vi "ECS - Scopes - DI4 Scope.vi"(11 "FPGA Ref":T1) -> ()   [LabVIEW 2015, in "ECS-RT.lvlib"]
uses:
  ECS-RT.lvlib
  Typedefs/FPGA Refs/Generic FPGA Ref.ctl
  <vilib>/Platform/TimedLoop/XDataNode/timing_clust.ctl
  <vilib>/Platform/TimedLoop/XDataNode/nitl_modes.ctl
  <vilib>/Platform/TimedLoop/XDataNode/wakeup.ctl
  <vilib>/Utility/error.llb/Error Cluster From Error Code.vi
  <vilib>/rvi/errors/niLvFpgaAdjustHostInterfaceError.vi
  Globals/DIScope Globals.vi
  <vilib>/rvi/interface/nirviReadWriteControl/nirviReadWriteControl.xnode
  <vilib>/Platform/TimedLoop/XDataNode/XDataNode.xnode
  <vilib>/Platform/TimedLoop/XDataNode/XDNodeRunTimeDep.lvlib
  <vilib>/rvi/interface/Simulation/niFpgaSimulationCallBeginRW.vi
  NiFpgaLv.dll
  ECS-Shared.lvlib
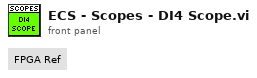
[diagram p1: front panel]
types:
  T1 = typedef "ECS-Shared.lvlib/Generic FPGA Ref.ctl" = refnum<k20>
  T2 = typedef "XDNodeRunTimeDep.lvlib/timing_clust.ctl" = cluster{"Expected End [f-1]":u64, "Actual End [f-1]":u64, "Finished Late? [f-1]":bool, "Expected End [i-1]":u64, "Actual End [i-1]":u64, "Finished Late? [i-1]":bool, "Expected Start [i]":u64, "Actual Start [i]":u64, "Expected Start [f]":u64, "Actual Start [f]":u64, "Source Name":string, "Structure Name":string, "Period":i64, "Deadline":i64, "Offset":i64, "Start":i64, "Priority":i32, "Timeout":i32, "Mode":T3, "Wakeup Reason":T4, "Error":errorcluster, "Source Type":string, "Secondary Source Type":string, "Global End Time":u64, "Global Start Time":u64, "Frame Duration":u64, "Iteration Duration":u64, "Assigned CPU":i32, "I/O Scan Engine Mode":u32}
  T3 = typedef "XDNodeRunTimeDep.lvlib/nitl_modes.ctl" = enum32{"No Change", "Process missed periods, maintain original phase", "Discard missed periods, maintain original phase", "Process missed periods, ignore original phase", "Discard missed periods, ignore original phase"}
  T4 = typedef "XDNodeRunTimeDep.lvlib/wakeup.ctl" = enum32{"Normal", "Aborted", "Asynchronous wakeup", "Timing source error", "Timed loop error", "Timeout"}
  T5 = cluster{"Element":u32, "Timed Out?":bool, "Elements Left":u32}
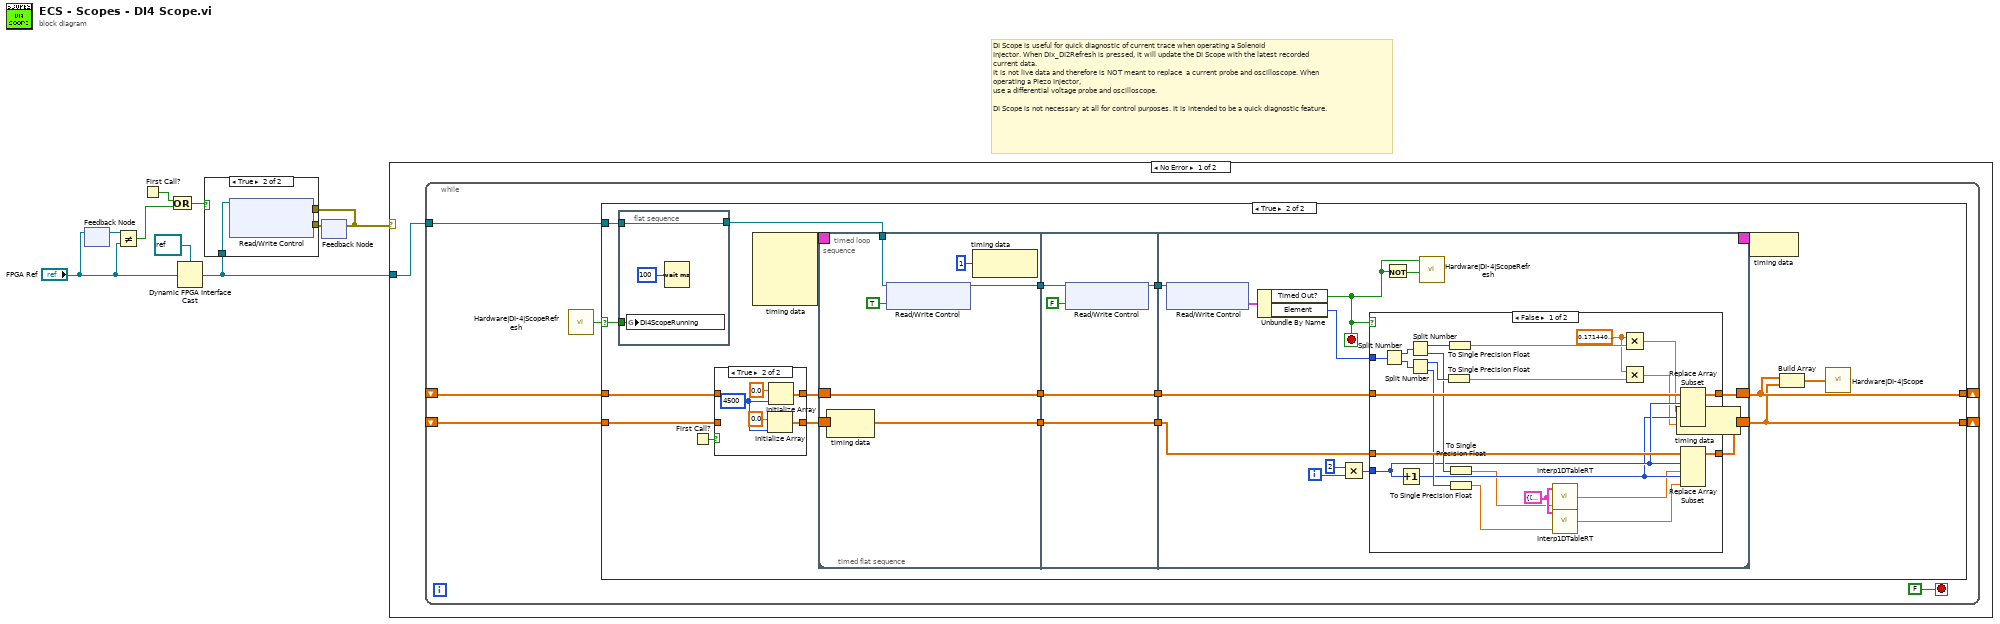
[diagram p0: block diagram]
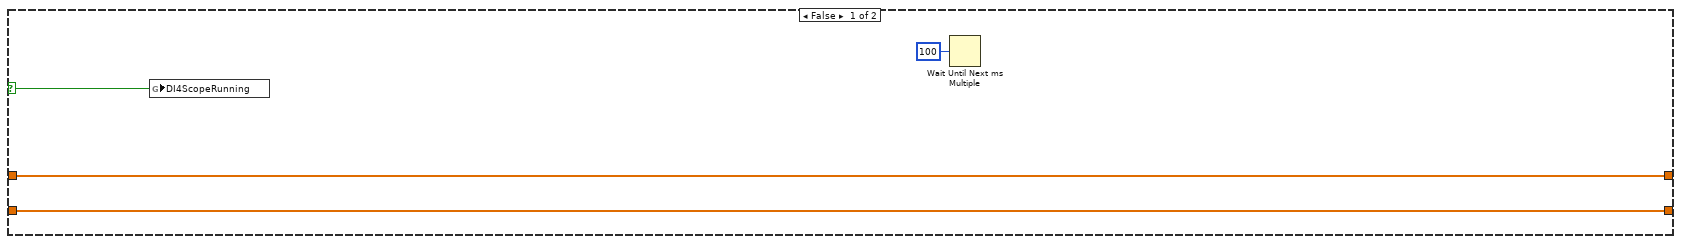
[diagram p3: hidden frame]
diagram:
  # "DI Scope is useful for quick diagnostic of current trace when operating a Solenoid\nInjector. When DIx_DI2Refresh is pressed, it will update the DI Scope with the latest recorded current data.\nIt is not live data and therefore is NOT meant to replace  a current probe and oscilloscope. When operating a Piezo Injector,\nuse a differential voltage probe and oscilloscope. \n\nDI Scope is not necessary at all for control purposes. It is intended to be a quick diagnostic feature."
  n1 = feedback #1() -> (w6:T1)  [unwired: 1 in]
  n2 = feedback-in #1("FPGA Ref") -> ()
  n3 = Not Equal?(x=w6, y="FPGA Ref") -> (x != y?=w5:bool)
  n4 = First Call?() -> (First Call?: T/F=w7:bool)
  n5 = Or(x=w7, y=w5) -> (x .or. y?=w8:bool)
  n6 = Dynamic FPGA Interface Cast(Session In=refnum<k20> refnum ("DI4 Scope"), Type="FPGA Ref") -> (Session Out=w3:refnum<k20>)
  n7 = feedback #2() -> (w9:errorcluster)  [unwired: 1 in]
  n8 = case shown="True" w8 {
    tunnel: [w10 w12] -> w4
    tunnel: w9 -> [w10 _]
    tunnel: w3 -> [_ w11]
    frame False {
    }
    frame True {
      n9 = xnode "Read/Write Control"("FPGA VI Reference In"=w11) -> ("error out"=w12:errorcluster)  [unwired: 2 in, 2 out]
    }
  }
  n10 = feedback-in #2(w4) -> ()
  n11 = case shown="No Error" w4 {
    tunnel: w3 -> [w13 _]
    frame No Error {
      n12 = while {
        shift-right: [w18] -> _
        shift-left: _ -> [w20]
        shift-right: [w17] -> _
        shift-left: _ -> [w19]
        tunnel: w13 -> [w16]
        stop <- FALSE stop-if-true
        n13 = call "Hardware|DI-4|ScopeRefresh"() -> ("Value"=w15:bool)
        n14 = case shown="True" w15 {
          selector: w15 -> [w22 w28]
          tunnel: w20 -> [w24 w35]
          tunnel: w19 -> [w23 w34]
          tunnel: [w24 w33] -> w18
          tunnel: [w23 w29] -> w17
          tunnel: w16 -> [_ w27]
          frame False {
            n15 = global write "DIScope Globals.vi" "DI4ScopeRunning"(w22) -> ()
            n16 = Wait Until Next ms Multiple(millisecond multiple=u32 100) -> ()  [unwired: 1 out]
          }
          frame True {
            n17 = flat-sequence {
              tunnel: w28 -> [w40]
              tunnel: [w38] -> w26
              tunnel: w27 -> [w38]
              frame #0 {
                n18 = global write "DIScope Globals.vi" "DI4ScopeRunning"(w40) -> ()
                n19 = Wait (ms)(milliseconds to wait=u32 100 ("millisecond multiple")) -> ()  [unwired: 1 out]
              }
            }
            n20 = First Call?() -> (First Call?: T/F=w37:bool)
            n21 = case shown="True" w37 {
              tunnel: [w118 w122] -> w36
              tunnel: [w117 w121] -> w32
              tunnel: w35 -> [w118 _]
              tunnel: w34 -> [w117 _]
              frame False {
              }
              frame True {
                w119 = 4500 ("dimension size")
                n22 = Initialize Array(sgl 0.0 ("element"), w119) -> (w121:sgl[])
                n23 = Initialize Array(sgl 0.0 ("element"), w119) -> (w122:sgl[])
              }
            }
            n24 = node-c288() -> (w31:T2)  [unwired: 4 in]
            n25 = timed-loop "Timed Loop" {
              shift-right: [w43] -> w33
              shift-left: w36 -> [w44]
              shift-right: [w41] -> w29
              shift-left: w32 -> [w42]
              tunnel: w26 -> [w45]
              timing: w31 -> [_]
              timing-out: [_] -> w30
              i -> [w77]
              stop <- w74 stop-if-true
              n26 = timed-sequence {
                timing: _ -> [_]
                timing-out: _ -> [_]
                tunnel: w45 -> [w56]
                tunnel: w44 -> [w55]
                tunnel: [w54] -> w43
                tunnel: w42 -> [w53]
                tunnel: [w52] -> w41
                n27 = timed-flat-sequence {
                  tunnel: w53 -> [w61]
                  tunnel: w55 -> [w62]
                  tunnel: w56 -> [w59]
                  tunnel: [w62] -> w49
                  tunnel: [w61] -> w48
                  tunnel: [w60] -> w47
                  tunnel: [w71] -> w51
                  tunnel: [w70] -> w50
                  tunnel: w47 -> [w68]
                  tunnel: w48 -> [w70]
                  tunnel: w49 -> [w71]
                  tunnel: [w67] -> w46
                  tunnel: [w82] -> w54
                  tunnel: [w81] -> w52
                  tunnel: w51 -> [w85]
                  tunnel: w50 -> [w84]
                  tunnel: w46 -> [w79]
                  frame #0 {
                    n28 = xnode "Read/Write Control"("FPGA VI Reference In"=w59, "DI-4.ScopeRead"=TRUE ("DIDI2Read")) -> ("FPGA VI Reference Out"=w60:refnum<k20>)  [unwired: 1 in, 1 out]
                    n29 = node-c288(i64 1 ("Start")) -> ()  [unwired: 1 out]
                  }
                  frame #1 {
                    n30 = xnode "Read/Write Control"("FPGA VI Reference In"=w68, "DI-4.ScopeRead"=FALSE ("DIDI2Read")) -> ("FPGA VI Reference Out"=w67:refnum<k20>)  [unwired: 1 in, 1 out]
                  }
                  frame #2 {
                    n31 = xnode "Read/Write Control"("FPGA VI Reference In"=w79) -> ("DI-4.ScopeData"=w80:T5)  [unwired: 1 in, 2 out]
                    n32 = Unbundle By Name(w80) -> ("Timed Out?"=w74:bool, "Element"=w76:u32)
                    n33 = Multiply(x=2, y=w77) -> (x*y=w78:i32)
                    n34 = case shown="False" w74 {
                      tunnel: w76 -> [w108 _]
                      tunnel: w85 -> [w105 w110]
                      tunnel: w84 -> [w104 w109]
                      tunnel: w78 -> [w97 _]
                      tunnel: [w99 w110] -> w82
                      tunnel: [w98 w109] -> w81
                      frame False {
                        w93 = sgl 0.17144 ("y")
                        w95 = cluster{"Counts (8bit)":sgl[], "Volts":sgl[]} {"Counts (8bit)"=[0.0, 26.0, 50.0, 74.0, 97.0, 120.0, 144.0, 167.0, 190.0, 213.0, 237.0], "Volts"=[0.0, 20.0, 40.0, 60.0, 80.0, 100.0, 120.0, 140.0, 160.0, 180.0, 200.0]} ("HVTable")
                        n35 = Split Number(x=w108) -> (hi(x)=w107:u16, lo(x)=w106:u16)
                        n36 = Increment(x=w97) -> (x+1=w96:i32)
                        n37 = Split Number(x=w107) -> (hi(x)=w101:u8, lo(x)=w100:u8)
                        n38 = Split Number(x=w106) -> (hi(x)=w103:u8, lo(x)=w102:u8)
                        n39 = To Single Precision Float(number=w103) -> (single precision float=w92:sgl)
                        n40 = To Single Precision Float(number=w101) -> (single precision float=w94:sgl)
                        n41 = To Single Precision Float(number=w100) -> (single precision float=w89:sgl)
                        n42 = To Single Precision Float(number=w102) -> (single precision float=w88:sgl)
                        n43 = call <vilib>:"Interp1DTableRT.vi"("X"=w89, "1DTable"=w95) -> ("Y"=w87:sgl)  [unwired: 1 in]
                        n44 = call <vilib>:"Interp1DTableRT.vi"("X"=w88, "1DTable"=w95) -> ("Y"=w86:sgl)  [unwired: 1 in]
                        n45 = Multiply(x=w93, y=w94) -> (x*y=w90:sgl)
                        n46 = Multiply(x=w93, y=w92) -> (x*y=w91:sgl)
                        n47 = Replace Array Subset(array=w105, new element #1=w90, index #1=w97, new element #2=w91, index #2=w96) -> (w99:sgl[])
                        n48 = Replace Array Subset(array=w104, new element #1=w87, index #1=w97, new element #2=w86, index #2=w96) -> (w98:sgl[])
                      }
                      frame True {
                      }
                    }
                    n49 = Not(x=w74) -> (.not. x?=w75:bool)
                    n50 = call "Hardware|DI-4|ScopeRefresh"("Value"=w75, "Adapt"=w74) -> ()  [unwired: 1 in]
                  }
                }
              }
              n51 = node-c288() -> ()  [unwired: 1 in, 1 out]
              n52 = node-c288() -> ()  [unwired: 1 in, 1 out]
            }
            n53 = node-c288(w30) -> ()
            n54 = Build Array(w33, w29) -> (w25:sgl[][])
            n55 = call "Hardware|DI-4|Scope"("Value"=w25) -> ()
          }
        }
      }
    }
    frame Error {
    }
  }
